vi "时间差（天）.vi"(9 "Start Time":timestamp, 11 "End Time":timestamp) -> (3 "Day":dbl)   [LabVIEW 2012]
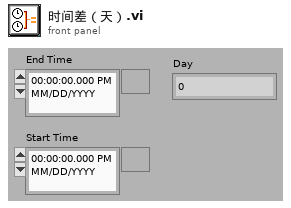
[diagram p1: front panel]
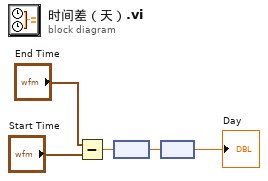
[diagram p0: block diagram]
diagram:
  n1 = Subtract(x="End Time", y="Start Time") -> (x-y=w3:dbl)
  n2 = node(w3) -> (w2:dbl[unit])
  n3 = node(w2) -> (→"Day":dbl)
